vi "I2C.vi"() -> ()   [LabVIEW 2019]
uses:
  <vilib>/myRIO/Instrument Drivers/Onboard IO/I2C/typedefs/I2C User Configuration.ctl
  <vilib>/myRIO/Instrument Drivers/Onboard IO/I2C/typedefs/I2C Transfer Rate.ctl
  <vilib>/myRIO/Instrument Drivers/Onboard IO/I2C/typedefs/I2C Reference.ctl
  <vilib>/myRIO/Common/Instrument Driver Framework/Utilities/typedefs/myRIO Generic Hardware Reference.ctl
  <vilib>/myRIO/Common/Instrument Driver Framework/Utilities/typedefs/Hardware Version Enum.ctl
  <vilib>/myRIO/Common/Instrument Driver Framework/Utilities/typedefs/myRIO v1.0 Reference.ctl
  <vilib>/myRIO/Common/Instrument Driver Framework/Utilities/typedefs/Generic FPGA Reference.ctl
  <vilib>/myRIO/Common/Instrument Driver Framework/myRIO v1.0/I2C/typedefs/I2C Channels Enum.ctl
  <vilib>/myRIO/Instrument Drivers/Onboard IO/I2C/typedefs/I2C Configuration.ctl
  <vilib>/userdefined/High Color/nirio_resource_hc.ctl
  <vilib>/myRIO/Common/Instrument Driver Framework/Utilities/vis/Is FPGA Ref Available.vi
  <vilib>/myRIO/Instrument Drivers/Onboard IO/I2C/vis/Configure.vi
  <vilib>/myRIO/Instrument Drivers/Onboard IO/I2C/vis/Write.vi
  <vilib>/myRIO/Instrument Drivers/Onboard IO/I2C/vis/Write Read.vi
  <vilib>/myRIO/Common/Instrument Driver Framework/Utilities/vis/Validate Channels.vi
  <vilib>/myRIO/Common/Instrument Driver Framework/myRIO v1.0/UART/vis/myRIO v1.0 Close UART.vi
  <vilib>/myRIO/Common/Instrument Driver Framework/ELVIS III v1.0/Resource Manager/vis/ELVIS III v1.0 Create Configuration List.vi
  <vilib>/Utility/VariantDataType/GetNumericInfo.vi
  <vilib>/Utility/error.llb/Error Cluster From Error Code.vi
  <vilib>/myRIO/Common/Instrument Driver Framework/ELVIS III v1.0/ELVIS III v1.1 Open.vi
  <vilib>/myRIO/Common/Instrument Driver Framework/ELVIS III v1.0/Resource Manager/vis/ELVIS III v1.0 Reserve Channel List.vi
  <vilib>/myRIO/Common/Instrument Driver Framework/ELVIS III v1.0/Resource Manager/vis/ELVIS III v1.0 Configure IO.vi
  <vilib>/myRIO/Common/Instrument Driver Framework/myRIO v1.0/myRIO v1.0 Close.vi
  <vilib>/myRIO/Common/Instrument Driver Framework/Utilities/vis/FPGA Ref Manager.vi
  <vilib>/myRIO/Common/Instrument Driver Framework/ELVIS III v1.0/ELVIS III v1.0 Reset FPGA.vi
  <vilib>/myRIO/Common/Instrument Driver Framework/myRIO v1.0/IRQ/vis/myRIO v1.0 IRQ Info FGV.vi
  <vilib>/myRIO/Common/Instrument Driver Framework/myRIO v1.0/IRQ/vis/myRIO v1.0 Timer IRQ Info FGV.vi
  <vilib>/myRIO/Common/Instrument Driver Framework/myRIO v1.0/IRQ/vis/myRIO v1.0 ISR Agent.vi
  <vilib>/myRIO/Instrument Drivers/Utilities/vis/Reset Index.vi
  <vilib>/myRIO/Common/Instrument Driver Framework/myRIO v1.0/Resource Manager/vis/myRIO v1.0 Block Write Resource Manager.vi
  <vilib>/myRIO/Express VI/Onboard IO/I2C/I2C Express VI.xnode
  <vilib>/myRIO/Instrument Drivers/Onboard IO/I2C/vis/myRIO I2C Open.xnode
  <vilib>/myRIO/Instrument Drivers/Utilities/Utilities.lvlib
  <vilib>/myRIO/Instrument Drivers/Onboard IO/I2C/I2C.lvlib
panel:
  out "Acceleration Data":T1(graph)={"Decimal Number Out"=0.14069369809477283, "Decimal Number Out"=0.9848558866634098, "Decimal Number Out"=0.14069369809477283}
  in  "Stop":bool
  out "Raw data":u8[](array[numeric]) format="%x"
  in  "Slave Address (7-bit)":u8=29 format="%x"
  # "ELVIS III Control IO"
  # "II2"
  # "Overview: Reads X, Y, and Z acceleration data from an MMA8452Q accelerometer.\nInstructions:\n1. Connect the MMA8452Q SDA, SCL, 3.3V, and GND lines to their respective Bank A ports (SDA - A/DIO15; SCL - A/DIO14).\n2. Supply power to the Application Board by pressing the button in the upper left corner of the NI ELVIS III.\n3. Run the VI."
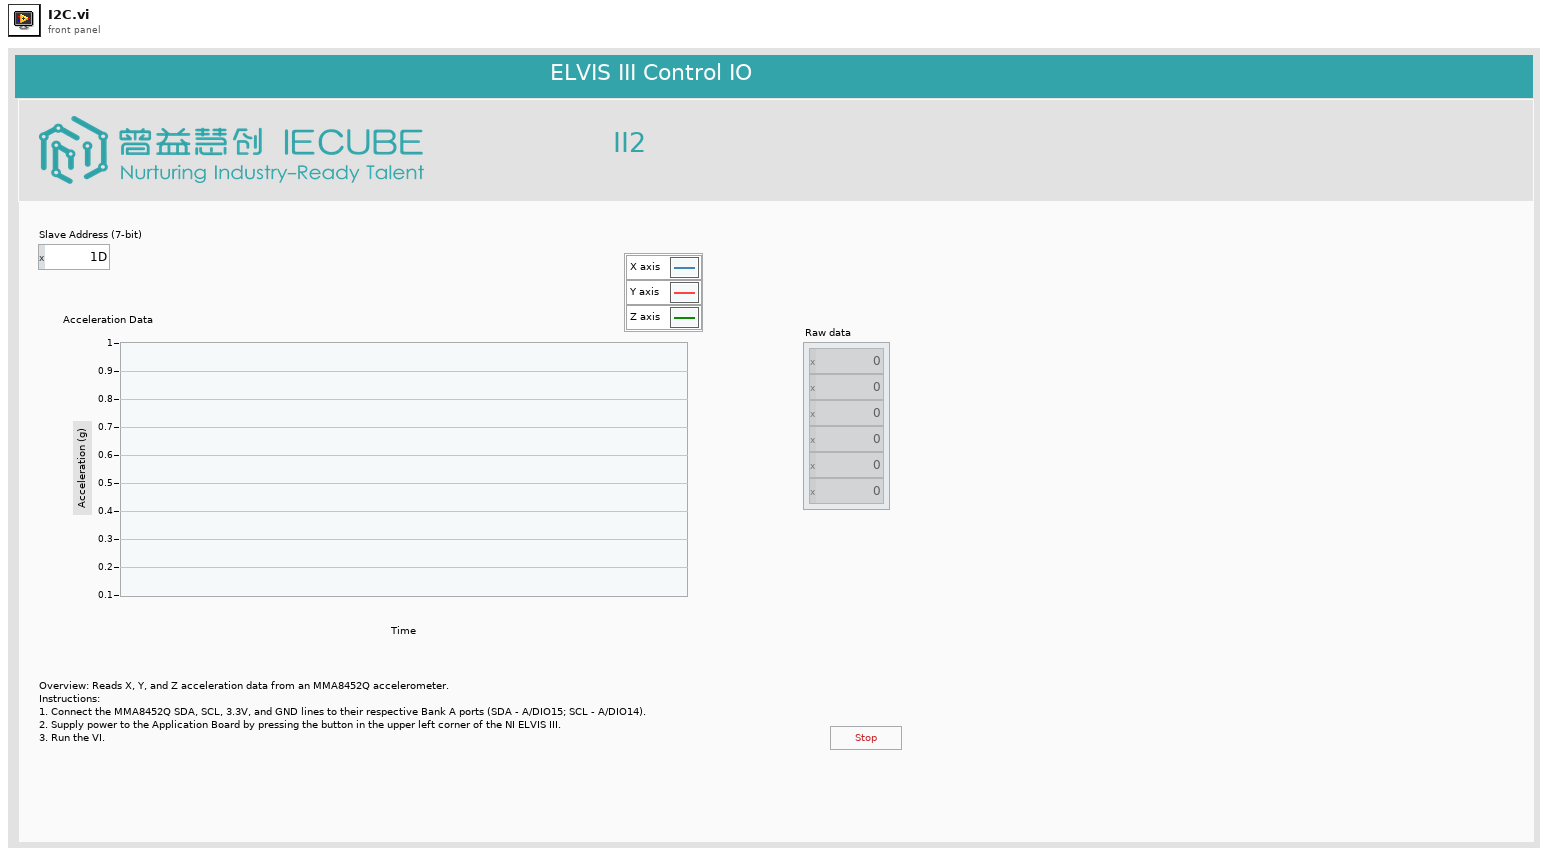
[diagram p1: front panel]
types:
  T1 = cluster{"Decimal Number Out":dbl, "Decimal Number Out":dbl, "Decimal Number Out":dbl}
  T2 = cluster{"Decimal Number Out":dbl, "Decimal Number Out":dbl, "Decimal Number Out":dbl}[]
  T3 = typedef "I2C.lvlib/I2C Reference.ctl" = cluster{"myRIO Reference":T4, "I2C Channels Enum":T8, "I2C Configuration":T9}
  T4 = typedef "myRIO Generic Hardware Reference.ctl" = cluster{"myRIO Model":T5, "myRIO Hardware Reference":T6}
  T5 = typedef "Hardware Version Enum.ctl" = enum16{"Unknown", "myRIO-1900", "myRIO-1950", "roboRIO", "NI ELVIS RIO CM", "ELVIS III"}
  T6 = typedef "myRIO v1.0 Reference.ctl" = cluster{"Generic FPGA Reference":T7, "Allow multiple opens":bool}
  T7 = typedef "Generic FPGA Reference.ctl" = refnum<k20>
  T8 = typedef "I2C Channels Enum.ctl" = enum16{"Not Connected", "A/I2C", "B/I2C", "I2C/I2C"}
  T9 = typedef "I2C.lvlib/I2C Configuration.ctl" = cluster{"I2C Transfer Rate":T10}
  T10 = typedef "I2C.lvlib/I2C Transfer Rate.ctl" = enum16{"Standard mode (100 kbps)", "Fast mode (400 kbps)"}
  T11 = typedef "I2C.lvlib/I2C User Configuration.ctl" = cluster{"I2C Transfer Rate":T10}
  T12 = typedef "nirio_resource_hc.ctl" = tag
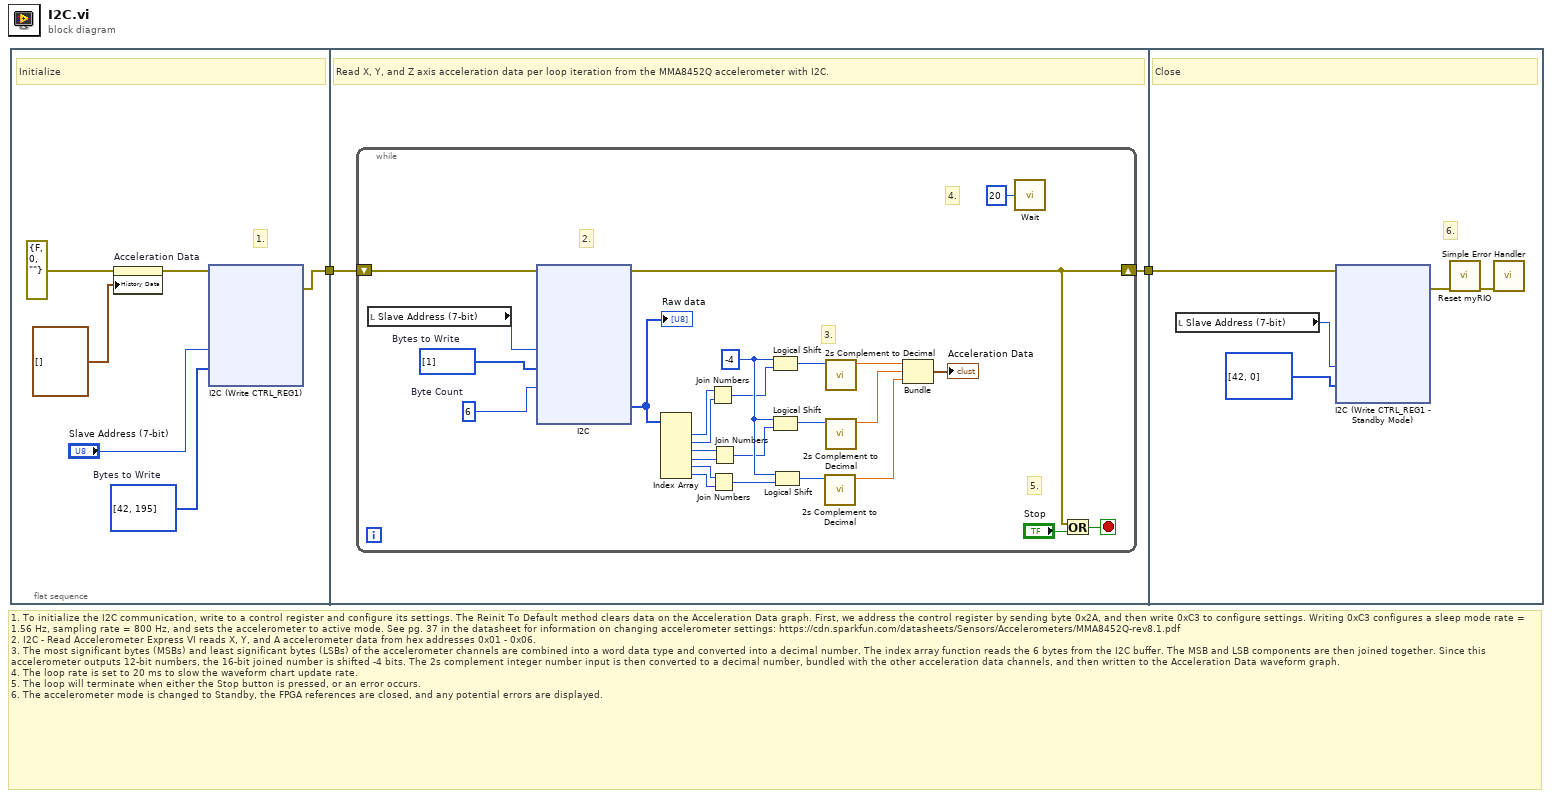
[diagram p0: block diagram]
diagram:
  # "1. To initialize the I2C communication, write to a control register and configure its settings. The Reinit To Default method clears data on the Acceleration Data graph. First, we address the control register by sending byte 0x2A, and then write 0xC3 to configure settings. Writing 0xC3 configures a sleep mode rate = 1.56 Hz, sampling rate = 800 Hz, and sets the accelerometer to active mode. See pg. 37 in the datasheet for information on changing accelerometer settings: https://cdn.sparkfun.com/datasheets/Sensors/Accelerometers/MMA8452Q-rev8.1.pdf\n2. I2C - Read Accelerometer Express VI reads X, Y, and A accelerometer data from hex addresses 0x01 - 0x06.\n3. The most significant bytes (MSBs) and least significant bytes (LSBs) of the accelerometer channels are combined into a word data type and converted into a decimal number. The index array function reads the 6 bytes from the I2C buffer. The MSB and LSB components are then joined together. Since this accelerometer outputs 12-bit numbers, the 16-bit joined number is shifted -4 bits. The 2s complement integer number input is then converted to a decimal number, bundled with the other acceleration data channels, and then written to the Acceleration Data waveform graph.\n4. The loop rate is set to 20 ms to slow the waveform chart update rate.\n5. The loop will terminate when either the Stop button is pressed, or an error occurs.\n6. The accelerometer mode is changed to Standby, the FPGA references are closed, and any potential errors are displayed."
  n1 = flat-sequence {
    tunnel: [w6] -> w2
    tunnel: w2 -> [w48]
    tunnel: [w47] -> w1
    tunnel: w1 -> [w117]
    frame #0 {
      w8 = u8[] [42, 195]  # Bytes to Write
      # "1."
      # "Initialize"
      n2 = property on="Acceleration Data" class="WFChart (严格)"(error in=errorcluster {"status"=FALSE, "code"=0, "source"=""} ("Error In"), "History Data"=T2 []) -> (error out=w3:errorcluster)  [unwired: 1 in, 1 out]
      n3 = xnode "I2C (Write CTRL_REG1)"("Slave Address (7-bit)"="Slave Address (7-bit)", "Bytes to Write"=w8, "error in (no error)"=w3) -> ("error out"=w6:errorcluster)
    }
    frame #1 {
      # "Read X, Y, and Z axis acceleration data per loop iteration from the MMA8452Q accelerometer with I2C."
      n4 = while {
        shift-right: [w58] -> w47
        shift-left: w48 -> [w59]
        stop <- w62 stop-if-true
        w61 = u32 6  # Byte Count
        w60 = u8[] [1]  # Bytes to Write
        w66 = i16 -4 ("y")
        # "5."
        # "4."
        # "3."
        # "2."
        n5 = local read "Slave Address (7-bit)"() -> (w55:u8)
        n6 = xnode "I2C"("Slave Address (7-bit)"=w55, "Bytes to Write"=w60, "Byte Count"=w61, "error in (no error)"=w59) -> ("Bytes Read"=w74:u8[], "error out"=w58:errorcluster)
        "Raw data" <- w74
        n7 = Index Array(array=w74) -> (element #1=w73:u8, element #2=w72:u8, element #3=w71:u8, element #4=w70:u8, element #5=w69:u8, element #6=w68:u8)  [unwired: 6 in]
        n8 = Join Numbers(hi=w73, lo=w72) -> ((hi.lo)=w63:u16)
        n9 = Join Numbers(hi=w69, lo=w68) -> ((hi.lo)=w65:u16)
        n10 = Join Numbers(hi=w71, lo=w70) -> ((hi.lo)=w64:u16)
        n11 = Logical Shift(y=w66, x=w63) -> (x << y=w57:u16)
        n12 = Logical Shift(y=w66, x=w64) -> (x << y=w56:u16)
        n13 = Logical Shift(y=w66, x=w65) -> (x << y=w49:u16)
        n14 = call "2s Complement to Decimal.vi"("2s Complement In"=w49) -> ("Decimal Number Out"=w52:dbl)  [unwired: 10 in]
        n15 = call "2s Complement to Decimal.vi"("2s Complement In"=w57) -> ("Decimal Number Out"=w54:dbl)  [unwired: 10 in]
        n16 = call "2s Complement to Decimal.vi"("2s Complement In"=w56) -> ("Decimal Number Out"=w53:dbl)  [unwired: 10 in]
        n17 = Bundle("Decimal Number Out"=w54, "Decimal Number Out"=w53, "Decimal Number Out"=w52) -> (→"Acceleration Data":T1)  [unwired: 1 in]
        n18 = call "Wait"("Count(mSec)"=u32 20) -> ()  [unwired: 1 out]
        n19 = Or(x=w58, y="Stop") -> (x .or. y?=w62:bool)
      }
    }
    frame #2 {
      # "6."
      # "Close"
      n20 = local read "Slave Address (7-bit)"() -> (w115:u8)
      n21 = xnode "I2C (Write CTRL_REG1 - Standby Mode)"("Slave Address (7-bit)"=w115, "Bytes to Write"=u8[] [42, 0], "error in (no error)"=w117) -> ("error out"=w116:errorcluster)
      n22 = call <vilib>:"Reset myRIO.vi"("error in (no error)"=w116) -> ("error out"=w119:errorcluster)  [unwired: 10 in]
      n23 = call <vilib>:"Simple Error Handler.vi"("error in (no error)"=w119) -> ()  [unwired: 4 in, 5 out]
    }
  }
